vi "MBUS_ReturnDataToTableEntry.vi"(10 "Exception Code":u8, 11 "dataIn":string) -> (3 "dataOut":string[](array[string]))   [LabVIEW 2012, in "MBUS_Modbus.lvlib"]
uses:
  MBUS_Modbus.lvlib
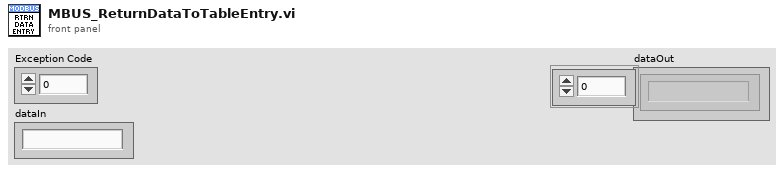
[diagram p1: front panel]
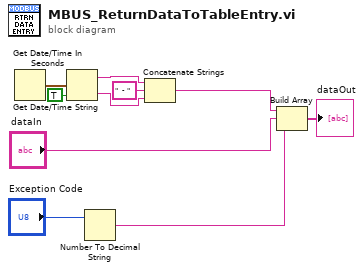
[diagram p0: block diagram]
diagram:
  n1 = Get Date/Time In Seconds() -> (seconds since 1Jan1904=w10:timestamp)
  n2 = Get Date/Time String(seconds (now)=w10, want seconds? (F)=TRUE) -> (date string=w7:string, time string=w6:string)  [unwired: 1 in]
  n3 = Number To Decimal String(number="Exception Code") -> (decimal integer string=w3:string)  [unwired: 1 in]
  n4 = Concatenate Strings(w7, "  - " ("string"), w6) -> (w5:string)
  n5 = Build Array(w5, "dataIn", w3) -> (→"dataOut":string[])
